vi "HHMMSS.vi"(11 "Time in Seconds":dbl) -> (0 "HH:MM:SS":string, 1 "Seconds":dbl, 2 "Mins":dbl, 3 "Hours":dbl)   [LabVIEW 2015]
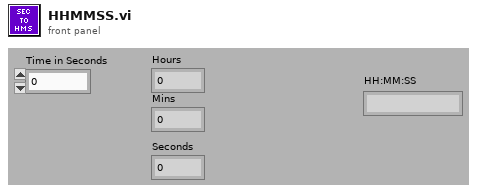
[diagram p1: front panel]
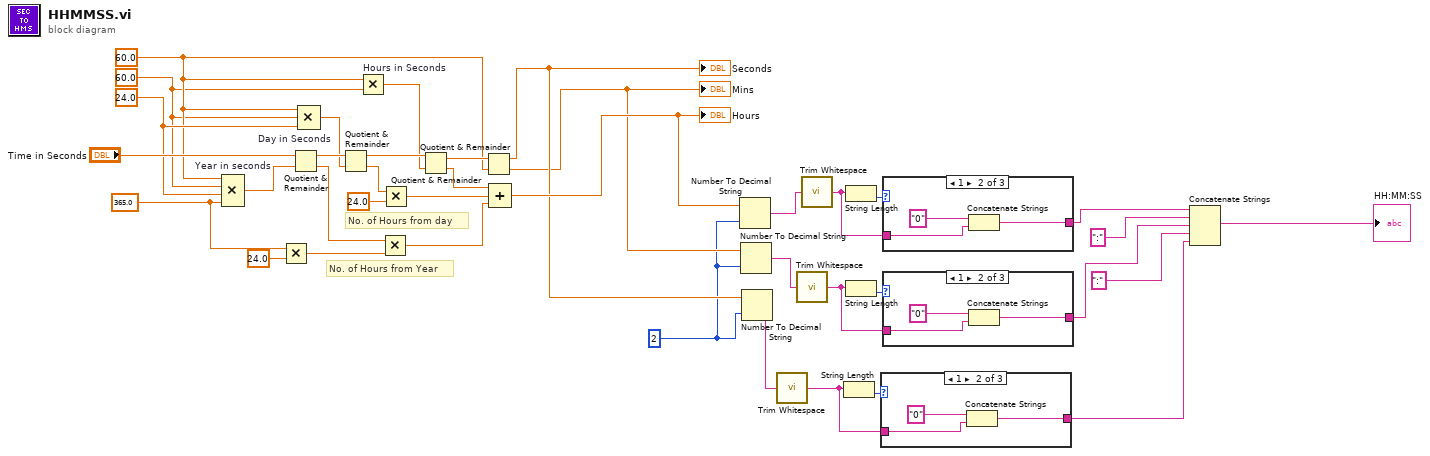
[diagram p0: block diagram]
diagram:
  w16 = 2
  w22 = 365.0
  w31 = 24.0
  w24 = 60.0
  w25 = 60.0
  # "No. of Hours from day"
  # "No. of Hours from Year"
  n1 = Compound Arithmetic op=MULTIPLY "Year in seconds"(w25, w24, w31, w22) -> (w37:dbl)
  n2 = Multiply(x=w22, y=24.0) -> (x*y=w20:dbl)
  n3 = Quotient & Remainder(x="Time in Seconds", y=w37) -> (x-y*floor(x/y)=w36:dbl, floor(x/y)=w33:dbl)
  n4 = Compound Arithmetic op=MULTIPLY "Day in Seconds"(w25, w24, w31) -> (w32:dbl)
  n5 = Quotient & Remainder(x=w36, y=w32) -> (x-y*floor(x/y)=w35:dbl, floor(x/y)=w30:dbl)
  n6 = Multiply "Hours in Seconds"(x=w25, y=w24) -> (x*y=w34:dbl)
  n7 = Multiply(x=w33, y=w20) -> (x*y=w26:dbl)
  n8 = Multiply(x=w30, y=24.0) -> (x*y=w27:dbl)
  n9 = Quotient & Remainder(x=w35, y=w34) -> (x-y*floor(x/y)=w29:dbl, floor(x/y)=w28:dbl)
  n10 = Quotient & Remainder(x=w29, y=w25) -> (x-y*floor(x/y)=w18:dbl, floor(x/y)=w17:dbl)
  "Mins" <- w17
  "Seconds" <- w18
  n11 = Compound Arithmetic op=ADD(w28, w27, w26) -> (w19:dbl)
  "Hours" <- w19
  n12 = Number To Decimal String(number=w19, width (-)=w16) -> (decimal integer string=w2:string)
  n13 = Number To Decimal String(number=w17, width (-)=w16) -> (decimal integer string=w6:string)
  n14 = Number To Decimal String(number=w18, width (-)=w16) -> (decimal integer string=w10:string)
  n15 = call <vilib>:"Trim Whitespace.vi"("string"=w10) -> ("trimmed string"=w9:string)  [unwired: 1 in]
  n16 = call <vilib>:"Trim Whitespace.vi"("string"=w6) -> ("trimmed string"=w7:string)  [unwired: 1 in]
  n17 = call <vilib>:"Trim Whitespace.vi"("string"=w2) -> ("trimmed string"=w3:string)  [unwired: 1 in]
  n18 = String Length(string=w9) -> (length=w12:i32)
  n19 = String Length(string=w3) -> (length=w4:i32)
  n20 = String Length(string=w7) -> (length=w8:i32)
  n21 = case shown="1" w12 {
    tunnel: w9 -> [w39 w42 w43]
    tunnel: [w39 w40 w43] -> w11
    frame 0, Default {
    }
    frame 1 {
      n22 = Concatenate Strings("0", w42) -> (w40:string)
    }
    frame 2 {
    }
  }
  n23 = case shown="1" w4 {
    tunnel: w3 -> [w44 w47 w48]
    tunnel: [w44 w45 w48] -> w1
    frame 0, Default {
    }
    frame 1 {
      n24 = Concatenate Strings("0", w47) -> (w45:string)
    }
    frame 2 {
    }
  }
  n25 = case shown="1" w8 {
    tunnel: w7 -> [w49 w52 w53]
    tunnel: [w49 w50 w53] -> w5
    frame 0, Default {
    }
    frame 1 {
      n26 = Concatenate Strings("0", w52) -> (w50:string)
    }
    frame 2 {
    }
  }
  n27 = Concatenate Strings(w1, ":", w5, ":", w11) -> (→"HH:MM:SS":string)
